vi "Waveform Chart, Set Cursors.vi"(6 "PosY":dbl=nan format="%.3p", 7 "PosX":dbl=nan format="%.3p", 8 "error in":errorcluster, 10 "cursor":u32, 11 "WFGraph ref":refnum<vi>) -> (0 "error out":errorcluster, 2 "next cursor":u32, 3 "WFGraph ref dup":refnum<vi>)   [LabVIEW 2010]
doc: "This function repositions the selected cursor on a waveform graph."
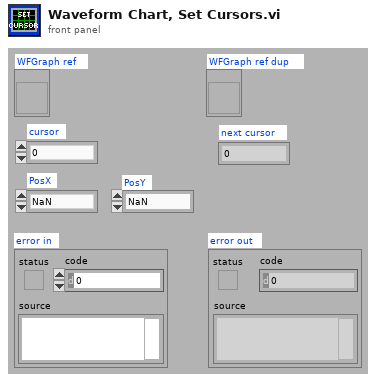
[diagram p1: front panel]
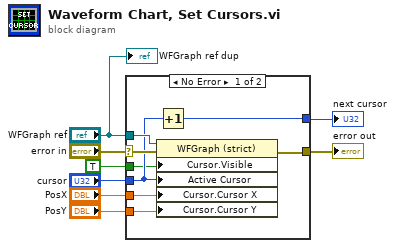
[diagram p0: block diagram]
diagram:
  n1 = case shown="No Error" "error in" {
    selector: "error in" -> [w15 w17]
    tunnel: [w14 w17] -> w7
    tunnel: "WFGraph ref" -> [w12 _]
    tunnel: "PosX" -> [w16 _]
    tunnel: "PosY" -> [w13 _]
    tunnel: "cursor" -> [w10 _]
    tunnel: [w11 _] -> w2
    tunnel: TRUE ("Cursor.Visible") -> [w9 _]
    frame No Error {
      n2 = property on="Property Node" class="WFGraph (strict)"(reference=w12, error in=w15, "Cursor.Visible"=w9, "Active Cursor"=w10, "Cursor.Cursor X"=w16, "Cursor.Cursor Y"=w13) -> (error out=w14:errorcluster)  [unwired: 1 out]
      n3 = Increment(x=w10) -> (x+1=w11:u32)
    }
    frame Error {
    }
  }
  "error out" <- w7
  "next cursor" <- w2
  "WFGraph ref dup" <- "WFGraph ref"
